vi "Get Component Settings.vi"(8 "error in (no error)":errorcluster, 10 "settings id":T1={"plugin"=-1, "thread"=-1, "group"=-1, "transfer"=-1, "channel"=-1}, 11 "framework configuration in":T4) -> (0 "error out":errorcluster, 2 "component settings":T2[](array[typedef]), 3 "framework configuration out":T4)   [LabVIEW 2017, in "DSF Core.lvlib"]
uses:
  DSF Core.lvlib
  Typedefs/DSF Engine Framework Configuration.ctl
  Typedefs/DSF Engine Plugin Configuration.ctl
  Typedefs/DSF Core Plugin Configuration.ctl
  Typedefs/DSF Timing Info.ctl
  Typedefs/DSF Settings Info.ctl
  Typedefs/DSF Version Info.ctl
  Typedefs/DSF Engine Plugin Thread Configuration.ctl
  Typedefs/DSF Core Thread Configuration.ctl
  Typedefs/DSF Engine Transfer Group Configuration.ctl
  Typedefs/DSF Core Group Configuration.ctl
  Typedefs/DSF Direction.ctl
  Typedefs/DSF Timeout Behavior.ctl
  Typedefs/DSF Engine Transfer Configuration.ctl
  Typedefs/DSF Core Transfer Configuration.ctl
  Typedefs/DSF Engine Channel Configuration.ctl
  Typedefs/DSF Core Channel Configuration.ctl
  Typedefs/DSF Data Type.ctl
  Typedefs/DSF Configuration ID.ctl
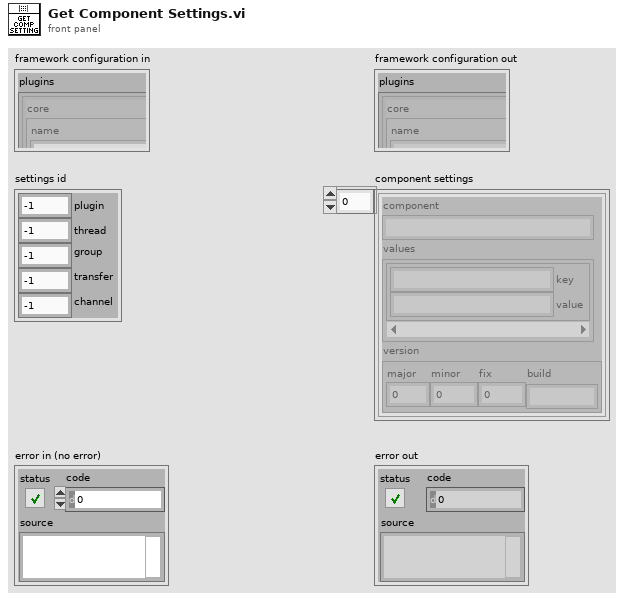
[diagram p1: front panel]
types:
  T1 = typedef "DSF Core.lvlib/DSF Configuration ID.ctl" = cluster{"plugin":i32, "thread":i32, "group":i32, "transfer":i32, "channel":i32}
  T2 = typedef "DSF Core.lvlib/DSF Settings Info.ctl" = cluster{"component":string, "values":cluster{"key":string, "value":string}[], "version":T3}
  T3 = typedef "DSF Core.lvlib/DSF Version Info.ctl" = cluster{"major":u32, "minor":u32, "fix":u32, "build":string}
  T4 = typedef "DSF Core.lvlib/DSF Engine Framework Configuration.ctl" = cluster{"plugins":T5[]}
  T5 = typedef "DSF Core.lvlib/DSF Engine Plugin Configuration.ctl" = cluster{"core":T6, "component settings":T2[], "threads":T8[]}
  T6 = typedef "DSF Core.lvlib/DSF Core Plugin Configuration.ctl" = cluster{"name":string, "components":string[], "cycle timing":T7}
  T7 = typedef "DSF Core.lvlib/DSF Timing Info.ctl" = cluster{"priority":u64, "decimation":u64, "offset":u64}
  T8 = typedef "DSF Core.lvlib/DSF Engine Plugin Thread Configuration.ctl" = cluster{"core":T9, "component settings":T2[], "transfer groups":T10[]}
  T9 = typedef "DSF Core.lvlib/DSF Core Thread Configuration.ctl" = cluster{"processor":i32, "priority offset":i16}
  T10 = typedef "DSF Core.lvlib/DSF Engine Transfer Group Configuration.ctl" = cluster{"core":T11, "component settings":T2[], "transfers":T14[]}
  T11 = typedef "DSF Core.lvlib/DSF Core Group Configuration.ctl" = cluster{"name":string, "direction":T12, "cycle timing":T7, "timeout behavior":T13}
  T12 = typedef "DSF Core.lvlib/DSF Direction.ctl" = enum8{"Tx", "Rx"}
  T13 = typedef "DSF Core.lvlib/DSF Timeout Behavior.ctl" = enum8{"Increment Late Count", "Throw Error"}
  T14 = typedef "DSF Core.lvlib/DSF Engine Transfer Configuration.ctl" = cluster{"core":T15, "component settings":T2[], "channels":T16[]}
  T15 = typedef "DSF Core.lvlib/DSF Core Transfer Configuration.ctl" = cluster{"name":string}
  T16 = typedef "DSF Core.lvlib/DSF Engine Channel Configuration.ctl" = cluster{"core":T17, "component settings":T2[]}
  T17 = typedef "DSF Core.lvlib/DSF Core Channel Configuration.ctl" = cluster{"name":string, "units":string, "engine data type":T18, "string data type":T18, "string offset":u64}
  T18 = typedef "DSF Core.lvlib/DSF Data Type.ctl" = enum8{"Bool", "SGL", "DBL", "I8", "I16", "I32", "I64", "U8", "U16", "U32", "U64"}
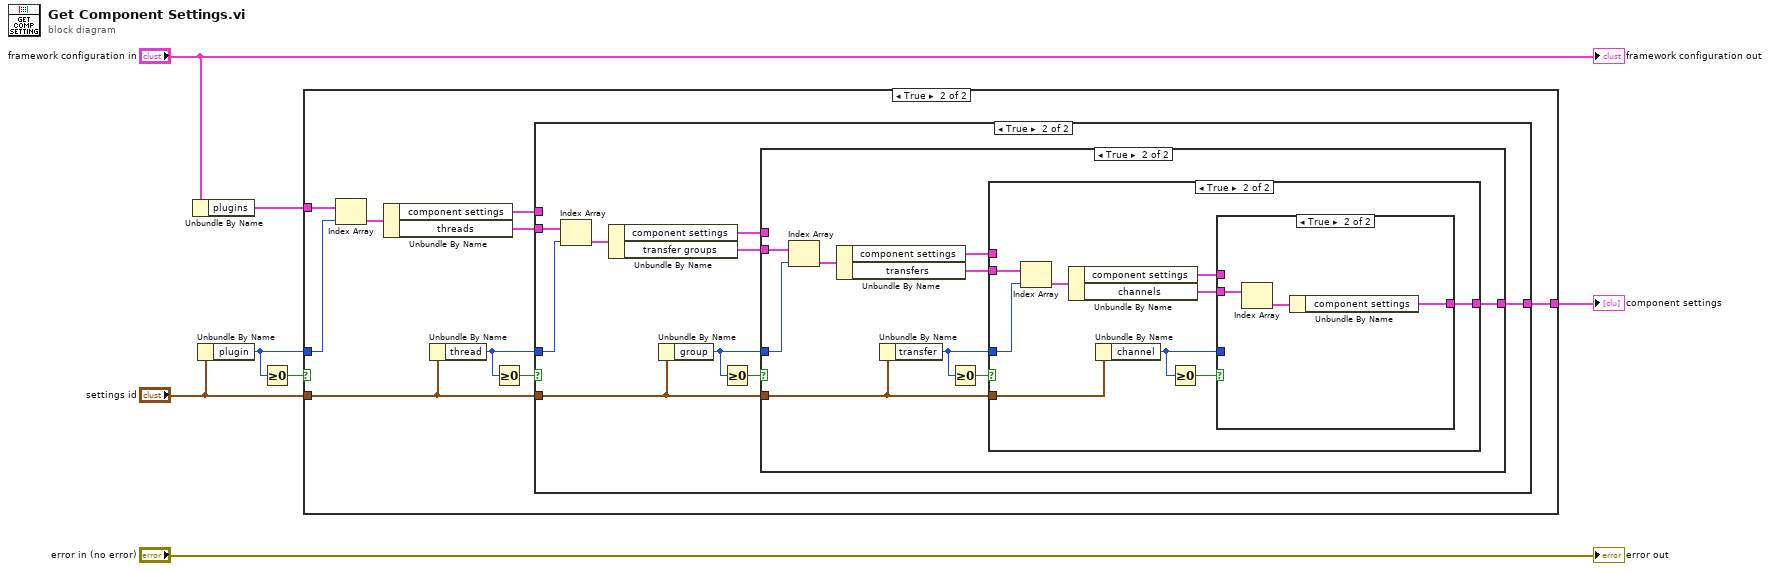
[diagram p0: block diagram]
diagram:
  n1 = Unbundle By Name("framework configuration in") -> ("plugins"=w5:T5[])
  n2 = Unbundle By Name("settings id") -> ("plugin"=w6:i32)
  n3 = Greater Or Equal To 0?(x=w6) -> (x >= 0?=w7:bool)
  n4 = case shown="True" w7 {
    tunnel: [_ w12] -> w1
    tunnel: "settings id" -> [_ w15]
    tunnel: w6 -> [_ w8]
    tunnel: w5 -> [_ w9]
    frame False {
    }
    frame True {
      n5 = Index Array(array=w9, index=w8) -> (element=w11:T5)
      n6 = Unbundle By Name(w11) -> ("component settings"=w13:T2[], "threads"=w10:T8[])
      n7 = Unbundle By Name(w15) -> ("thread"=w14:i32)
      n8 = Greater Or Equal To 0?(x=w14) -> (x >= 0?=w16:bool)
      n9 = case shown="True" w16 {
        tunnel: w15 -> [_ w26]
        tunnel: w14 -> [_ w19]
        tunnel: w13 -> [w17 _]
        tunnel: [w17 w20] -> w12
        tunnel: w10 -> [_ w22]
        frame False {
        }
        frame True {
          n10 = Index Array(array=w22, index=w19) -> (element=w23:T8)
          n11 = Unbundle By Name(w23) -> ("component settings"=w21:T2[], "transfer groups"=w18:T10[])
          n12 = Unbundle By Name(w26) -> ("group"=w24:i32)
          n13 = Greater Or Equal To 0?(x=w24) -> (x >= 0?=w25:bool)
          n14 = case shown="True" w25 {
            tunnel: w26 -> [_ w36]
            tunnel: w24 -> [_ w31]
            tunnel: w21 -> [w27 _]
            tunnel: [w27 w28] -> w20
            tunnel: w18 -> [_ w32]
            frame False {
            }
            frame True {
              n15 = Index Array(array=w32, index=w31) -> (element=w33:T10)
              n16 = Unbundle By Name(w33) -> ("component settings"=w29:T2[], "transfers"=w30:T14[])
              n17 = Unbundle By Name(w36) -> ("transfer"=w34:i32)
              n18 = Greater Or Equal To 0?(x=w34) -> (x >= 0?=w35:bool)
              n19 = case shown="True" w35 {
                tunnel: w36 -> [_ w46]
                tunnel: w34 -> [_ w41]
                tunnel: w30 -> [_ w42]
                tunnel: w29 -> [w37 _]
                tunnel: [w37 w38] -> w28
                frame False {
                }
                frame True {
                  n20 = Index Array(array=w42, index=w41) -> (element=w43:T14)
                  n21 = Unbundle By Name(w43) -> ("component settings"=w39:T2[], "channels"=w40:T16[])
                  n22 = Unbundle By Name(w46) -> ("channel"=w44:i32)
                  n23 = Greater Or Equal To 0?(x=w44) -> (x >= 0?=w45:bool)
                  n24 = case shown="True" w45 {
                    tunnel: w44 -> [_ _]
                    tunnel: w40 -> [_ w49]
                    tunnel: w39 -> [w47 _]
                    tunnel: [w47 w48] -> w38
                    frame False {
                    }
                    frame True {
                      n25 = Index Array(array=w49) -> (element=w50:T16)  [unwired: 1 in]
                      n26 = Unbundle By Name(w50) -> ("component settings"=w48:T2[])
                    }
                  }
                }
              }
            }
          }
        }
      }
    }
  }
  "component settings" <- w1
  "framework configuration out" <- "framework configuration in"
  "error out" <- "error in (no error)"
